vi "svx_Check Segment (Rev) vi.vi"(7 "reset in":bool, 8 "error in (no error)":errorcluster, 11 "segment settings":cluster{"start [rev]":dbl, "end [rev]":dbl}) -> (0 "error out":errorcluster, 3 "actual segment settings":cluster{"start [rev]":dbl, "end [rev]":dbl}={"start [rev]"=0.0, "end [rev]"=inf}, 5 "reset out":bool)   [LabVIEW 2017]
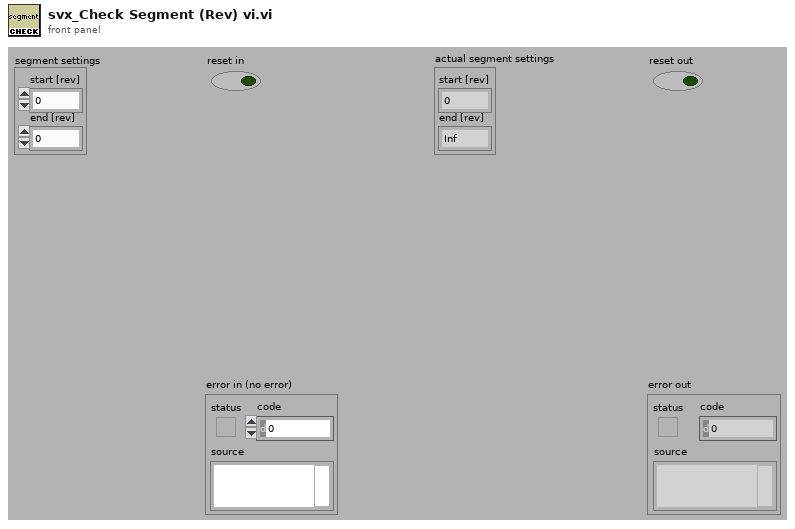
[diagram p1: front panel]
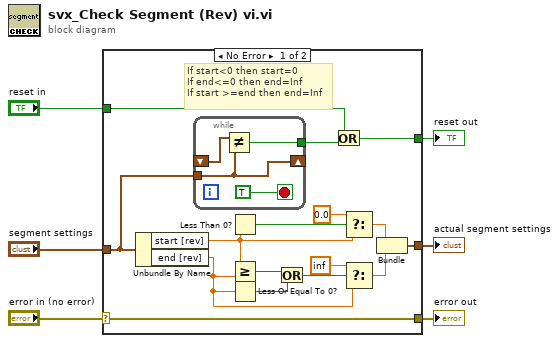
[diagram p0: block diagram]
diagram:
  n1 = case shown="No Error" "error in (no error)" {
    selector: "error in (no error)" -> [w22 w27]
    tunnel: "segment settings" -> [w10 _]
    tunnel: [w22 w27] -> w4
    tunnel: [w21 _] -> w3
    tunnel: "reset in" -> [w8 _]
    tunnel: [w7 _] -> w1
    frame No Error {
      # "If start<0 then start=0\nIf end<=0 then end=Inf\nIf start >=end then end=Inf"
      n2 = Unbundle By Name(w10) -> ("start [rev]"=w14:dbl, "end [rev]"=w11:dbl)
      n3 = while {
        tunnel: w10 -> [w24]
        shift-right: [w24] -> _
        shift-left: _ -> [w25]
        tunnel: [w23] -> w9
        stop <- TRUE stop-if-true
        n4 = Not Equal?(x=w25, y=w24) -> (x != y?=w23:bool)
      }
      n5 = Less Than 0?(x=w14) -> (x < 0?=w15:bool)
      n6 = Greater Or Equal?(x=w14, y=w11) -> (x >= y?=w20:bool)
      n7 = Less Or Equal To 0?(x=w11) -> (x <= 0?=w18:bool)
      n8 = Or(x=w20, y=w18) -> (x .or. y?=w19:bool)
      n9 = Or(x=w8, y=w9) -> (x .or. y?=w7:bool)
      n10 = Select(t=0.0, s=w15, f=w14) -> (s? t:f=w12:dbl)
      n11 = Select(t=inf ("f"), s=w19, f=w11) -> (s? t:f=w13:dbl)
      n12 = Bundle("start [rev]"=w12, "end [rev]"=w13) -> (w21:cluster{"start [rev]":dbl, "end [rev]":dbl})  [unwired: 1 in]
    }
    frame Error {
    }
  }
  "error out" <- w4
  "actual segment settings" <- w3
  "reset out" <- w1
